vi "ImportLaser.vi"(8 "error in (no error)":errorcluster, 9 "reference":refnum<vi>, 10 "laser":T1, 11 "Database in":refnum<class "Database.lvclass">) -> (0 "error out":errorcluster, 1 "reference 2":refnum<vi>, 3 "Database out":refnum<class "Database.lvclass">)   [LabVIEW 2014, in "Database.lvclass"]
uses:
  Database.lvclass
  Database.lvclass/Database.ctl
  <vilib>/addons/database/NI_Database_API.lvlib
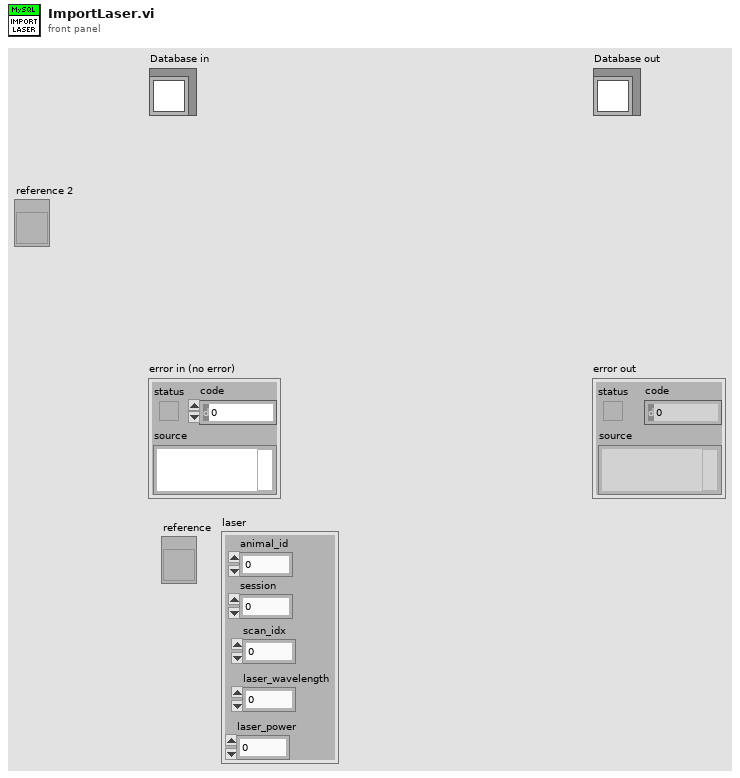
[diagram p1: front panel]
types:
  T1 = cluster{"animal_id":dbl, "session":dbl, "scan_idx":dbl, "laser_wavelength":dbl, "laser_power":dbl}
  T2 = typedef "NI_Database_API.lvlib/Conn ObjectReference.ctl" = refnum<k1>
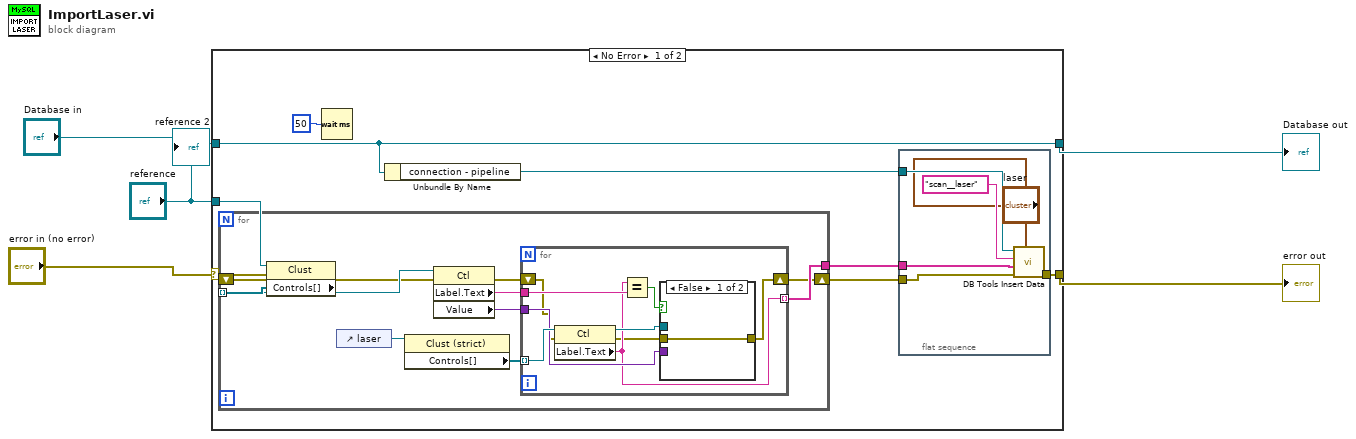
[diagram p0: block diagram]
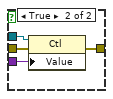
[diagram p2: hidden frame]
diagram:
  n1 = case shown="No Error" "error in (no error)" {
    selector: "error in (no error)" -> [w9 w46]
    tunnel: [w7 w46] -> w4
    tunnel: [w8 w45] -> w2
    tunnel: "Database in" -> [w8 w45]
    tunnel: "reference" -> [w6 _]
    frame No Error {
      n2 = property class="Clust"(reference=w6, error in=w9) -> (error out=w14:errorcluster, "Controls[]"=w15:refnum<vi>[])  [unwired: 1 out]
      n3 = for {
        tunnel: w15 -> [w30] mode=indexing
        shift-right: [w22] -> w11
        shift-left: w14 -> [w29]
        tunnel: [w27] -> w13
        n4 = control-ref of="laser"() -> (w28:refnum<vi>)
        n5 = property class="Clust (strict)"(reference=w28) -> ("Controls[]"=w26:refnum<vi>[])  [unwired: 1 in, 2 out]
        n6 = property class="Ctl"(reference=w30, error in=w29) -> (error out=w25:errorcluster, "Label.Text"=w23:string, "Value"=w24:variant)  [unwired: 1 out]
        n7 = for {
          tunnel: w23 -> [w39]
          tunnel: w24 -> [w36]
          tunnel: w26 -> [w38] mode=indexing
          tunnel: [w34] -> w27 mode=indexing
          shift-right: [w32] -> w22
          shift-left: w25 -> [w31]
          n8 = property class="Ctl"(reference=w38, error in=w31) -> (reference out=w37:refnum<vi>, error out=w33:errorcluster, "Label.Text"=w34:string)
          n9 = Equal?(x=w34, y=w39) -> (x = y?=w35:bool)
          n10 = case shown="False" w35 {
            tunnel: w37 -> [_ w44]
            tunnel: w36 -> [_ w43]
            tunnel: w33 -> [w40 w42]
            tunnel: [w40 w41] -> w32
            frame False {
            }
            frame True {
              n11 = property class="Ctl"(reference=w44, error in=w42, "Value"=w43) -> (error out=w41:errorcluster)  [unwired: 1 out]
            }
          }
        }
      }
      n12 = Wait (ms)(milliseconds to wait=u32 50) -> ()  [unwired: 1 out]
      n13 = Unbundle By Name(w8) -> ("connection - pipeline"=w12:T2)
      n14 = flat-sequence {
        tunnel: w13 -> [w21]
        tunnel: w12 -> [w20]
        tunnel: w11 -> [w19]
        tunnel: [w17] -> w7
        frame #0 {
          n15 = call <vilib>:"DB Tools Insert Data.vi"("data"="laser", "error in (no error)"=w19, "columns"=w21, "table"="scan__laser" ("session"), "connection reference"=w20) -> ("error out"=w17:errorcluster)  [unwired: 5 in, 1 out]
        }
      }
    }
    frame Error {
    }
  }
  "error out" <- w4
  "Database out" <- w2
  "reference 2" <- "reference"
